vi "Stop Core.vi"(10 "final error code":i32, 11 "Main View in":refnum<class "Main View.lvclass">) -> (3 "Main View out":refnum<class "Main View.lvclass">)   [LabVIEW 2013, in "Main View.lvlib" / "Main View.lvclass"]
doc: "(<B>Filename</B>: Actor Framework.lvlib:Actor.lvclass:Stop Core.vi)\n\nDefines what the actor does before it stops. Use the <B>final error code</B> input to determine whether the actor shut down in response to an error.\n\nBy default, this method does nothing. A descendant class may override it to define behavior, such as shutting down any processes the actor initiated in its override of the Actor Core method."
uses:
  Main View.lvclass
  <vilib>/ActorFrameworkMVC/View Actor/View Actor.lvclass
  Main View.lvclass/Main View.ctl
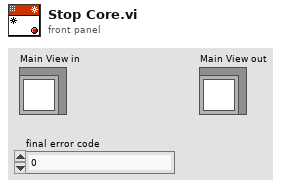
[diagram p1: front panel]
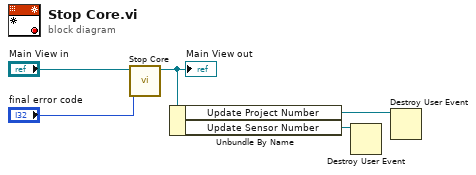
[diagram p0: block diagram]
diagram:
  n1 = call-parent "Stop Core.vi"("final error code"="final error code", "Actor in"="Main View in") -> ("Actor out"=w2:refnum<class "Main View.lvclass">)  [unwired: 9 in]
  "Main View out" <- w2
  n2 = Unbundle By Name(w2) -> ("Update Project Number"=w4:refnum<user-event>, "Update Sensor Number"=w1:refnum<user-event>)
  n3 = Destroy User Event(user event=w1) -> ()  [unwired: 1 in, 1 out]
  n4 = Destroy User Event(user event=w4) -> ()  [unwired: 1 in, 1 out]
